vi "solar_qtimer Refnum QTimer to SEQ.vi"(1 "QTimer Refnum":T1) -> (0 "QTimers SEQ":refnum<queue>)   [LabVIEW 2018]
doc: "This type casts from the Voyager reference."
uses:
  solar_qtimer_ctl QTimer.ctl
  solar_qtimer_ctl SEQ.ctl
  solar_qtimer_ctl QTimer Settings.ctl
  solar_qtimer_ctl Refnum.ctl
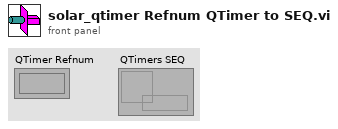
[diagram p1: front panel]
types:
  T1 = typedef "solar_qtimer_ctl Refnum.ctl" = refnum<k1>
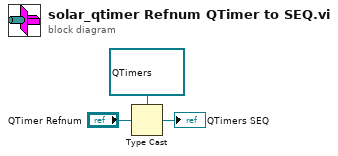
[diagram p0: block diagram]
diagram:
  n1 = Type Cast(type=refnum<queue> refnum ("QTimers SEQ"), x="QTimer Refnum") -> (*(type *) &x=→"QTimers SEQ":refnum<queue>)
